vi "Set Color.vi"(8 "error in (no error)":errorcluster, 10 "Color":u32(colorbox), 11 "Style in":refnum<class "Style.lvclass">) -> (0 "error out":errorcluster, 3 "Style out":refnum<class "Style.lvclass">)   [LabVIEW 2017, in "Styles.lvlib" / "Style.lvclass"]
uses:
  Style.lvclass
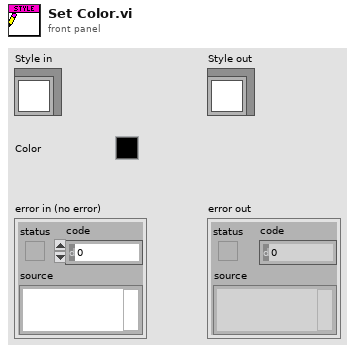
[diagram p1: front panel]
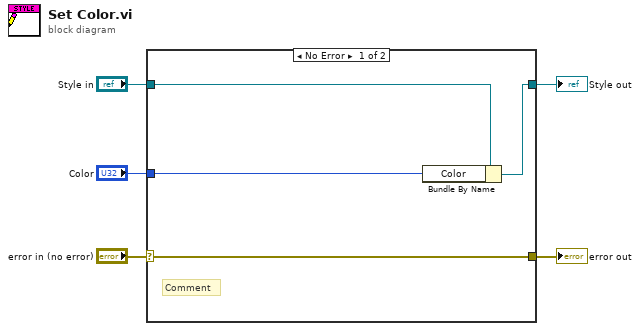
[diagram p0: block diagram]
diagram:
  n1 = case shown="No Error" "error in (no error)" {
    selector: "error in (no error)" -> [w9 w10]
    tunnel: [w9 w10] -> w4
    tunnel: [w7 w11] -> w2
    tunnel: "Style in" -> [w8 w11]
    tunnel: "Color" -> [w6 _]
    frame No Error {
      # "Comment"
      n2 = Bundle By Name(cluster=w8, "Color"=w6) -> (w7:refnum<class "Style.lvclass">)
    }
    frame Error {
    }
  }
  "error out" <- w4
  "Style out" <- w2
